vi "calibr_table.vi"() -> ()   [LabVIEW 2010]
panel:
  in  "Array":cluster{"Uin":dbl[], "ADCode":dbl[]}[](array[cluster]) {"ADCode" format="%.1f"; "Uin" format="%^_4g"}
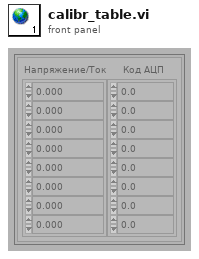
[diagram p1: front panel]
diagram:
